vi "Counter+AOtest.vi"() -> ()   [LabVIEW 2010]
uses:
  <vilib>/DAQmx/write.llb/DAQmx Write (Analog 2D DBL NChan NSamp).vi
  <vilib>/DAQmx/read.llb/DAQmx Read (Counter 1D U32 1Chan NSamp).vi
  <vilib>/DAQmx/create/channels.llb/DAQmx Create Channel (CI-Count Edges).vi
  <vilib>/DAQmx/configure/timing.llb/DAQmx Timing (Sample Clock).vi
  <vilib>/DAQmx/create/channels.llb/DAQmx Create Channel (AO-Voltage-Basic).vi
  <vilib>/daqmx/miscellaneous.llb/DAQmx Fill In Error Info.vi
  Program Files/National Instruments/LabVIEW 2010/resource/objmgr/daqmx.rc
panel:
  out "counter 1":u32[](graph)
  out "counter 2":u32[](graph)
  out "Y waveform":dbl[](graph)
  out "X waveform":dbl[](graph)
  out "error out AO":errorcluster
  out "task out AO":refnum<k21>
  out "error out CH1":errorcluster
  out "error out CH2":errorcluster
  out "Task CI CH2":refnum<k21>
  out "Task CI CH1":refnum<k21>
  in  "Field Size(V)":i8=1 caption="x-res" min=0 max=10
  out "P":dbl
  out "AI number of scans":i32=423936
  out "bin value":u32=1 caption="length [ms]" min=1 max=8 step=1
  in  "AI rate":u32=100000
  out "y-res new":i32=128
  out "x-res new":i32=128 caption="x-res new]"
  in  "resolution":u16(ring)=512 items=["128x"=128, "256x"=256, "512x"=512, "1024x"=1024]
  in  "x-res":i32=128
  in  "y-res":i32=128 caption="y-res]"
  in  "quick res":bool caption="quick"
  out "Y-WaveArray":dbl[](array[numeric])
  out "X-WaveArray":dbl[](array[numeric])
  out "numPixels":dbl
  in  "AO rate":u32=100000
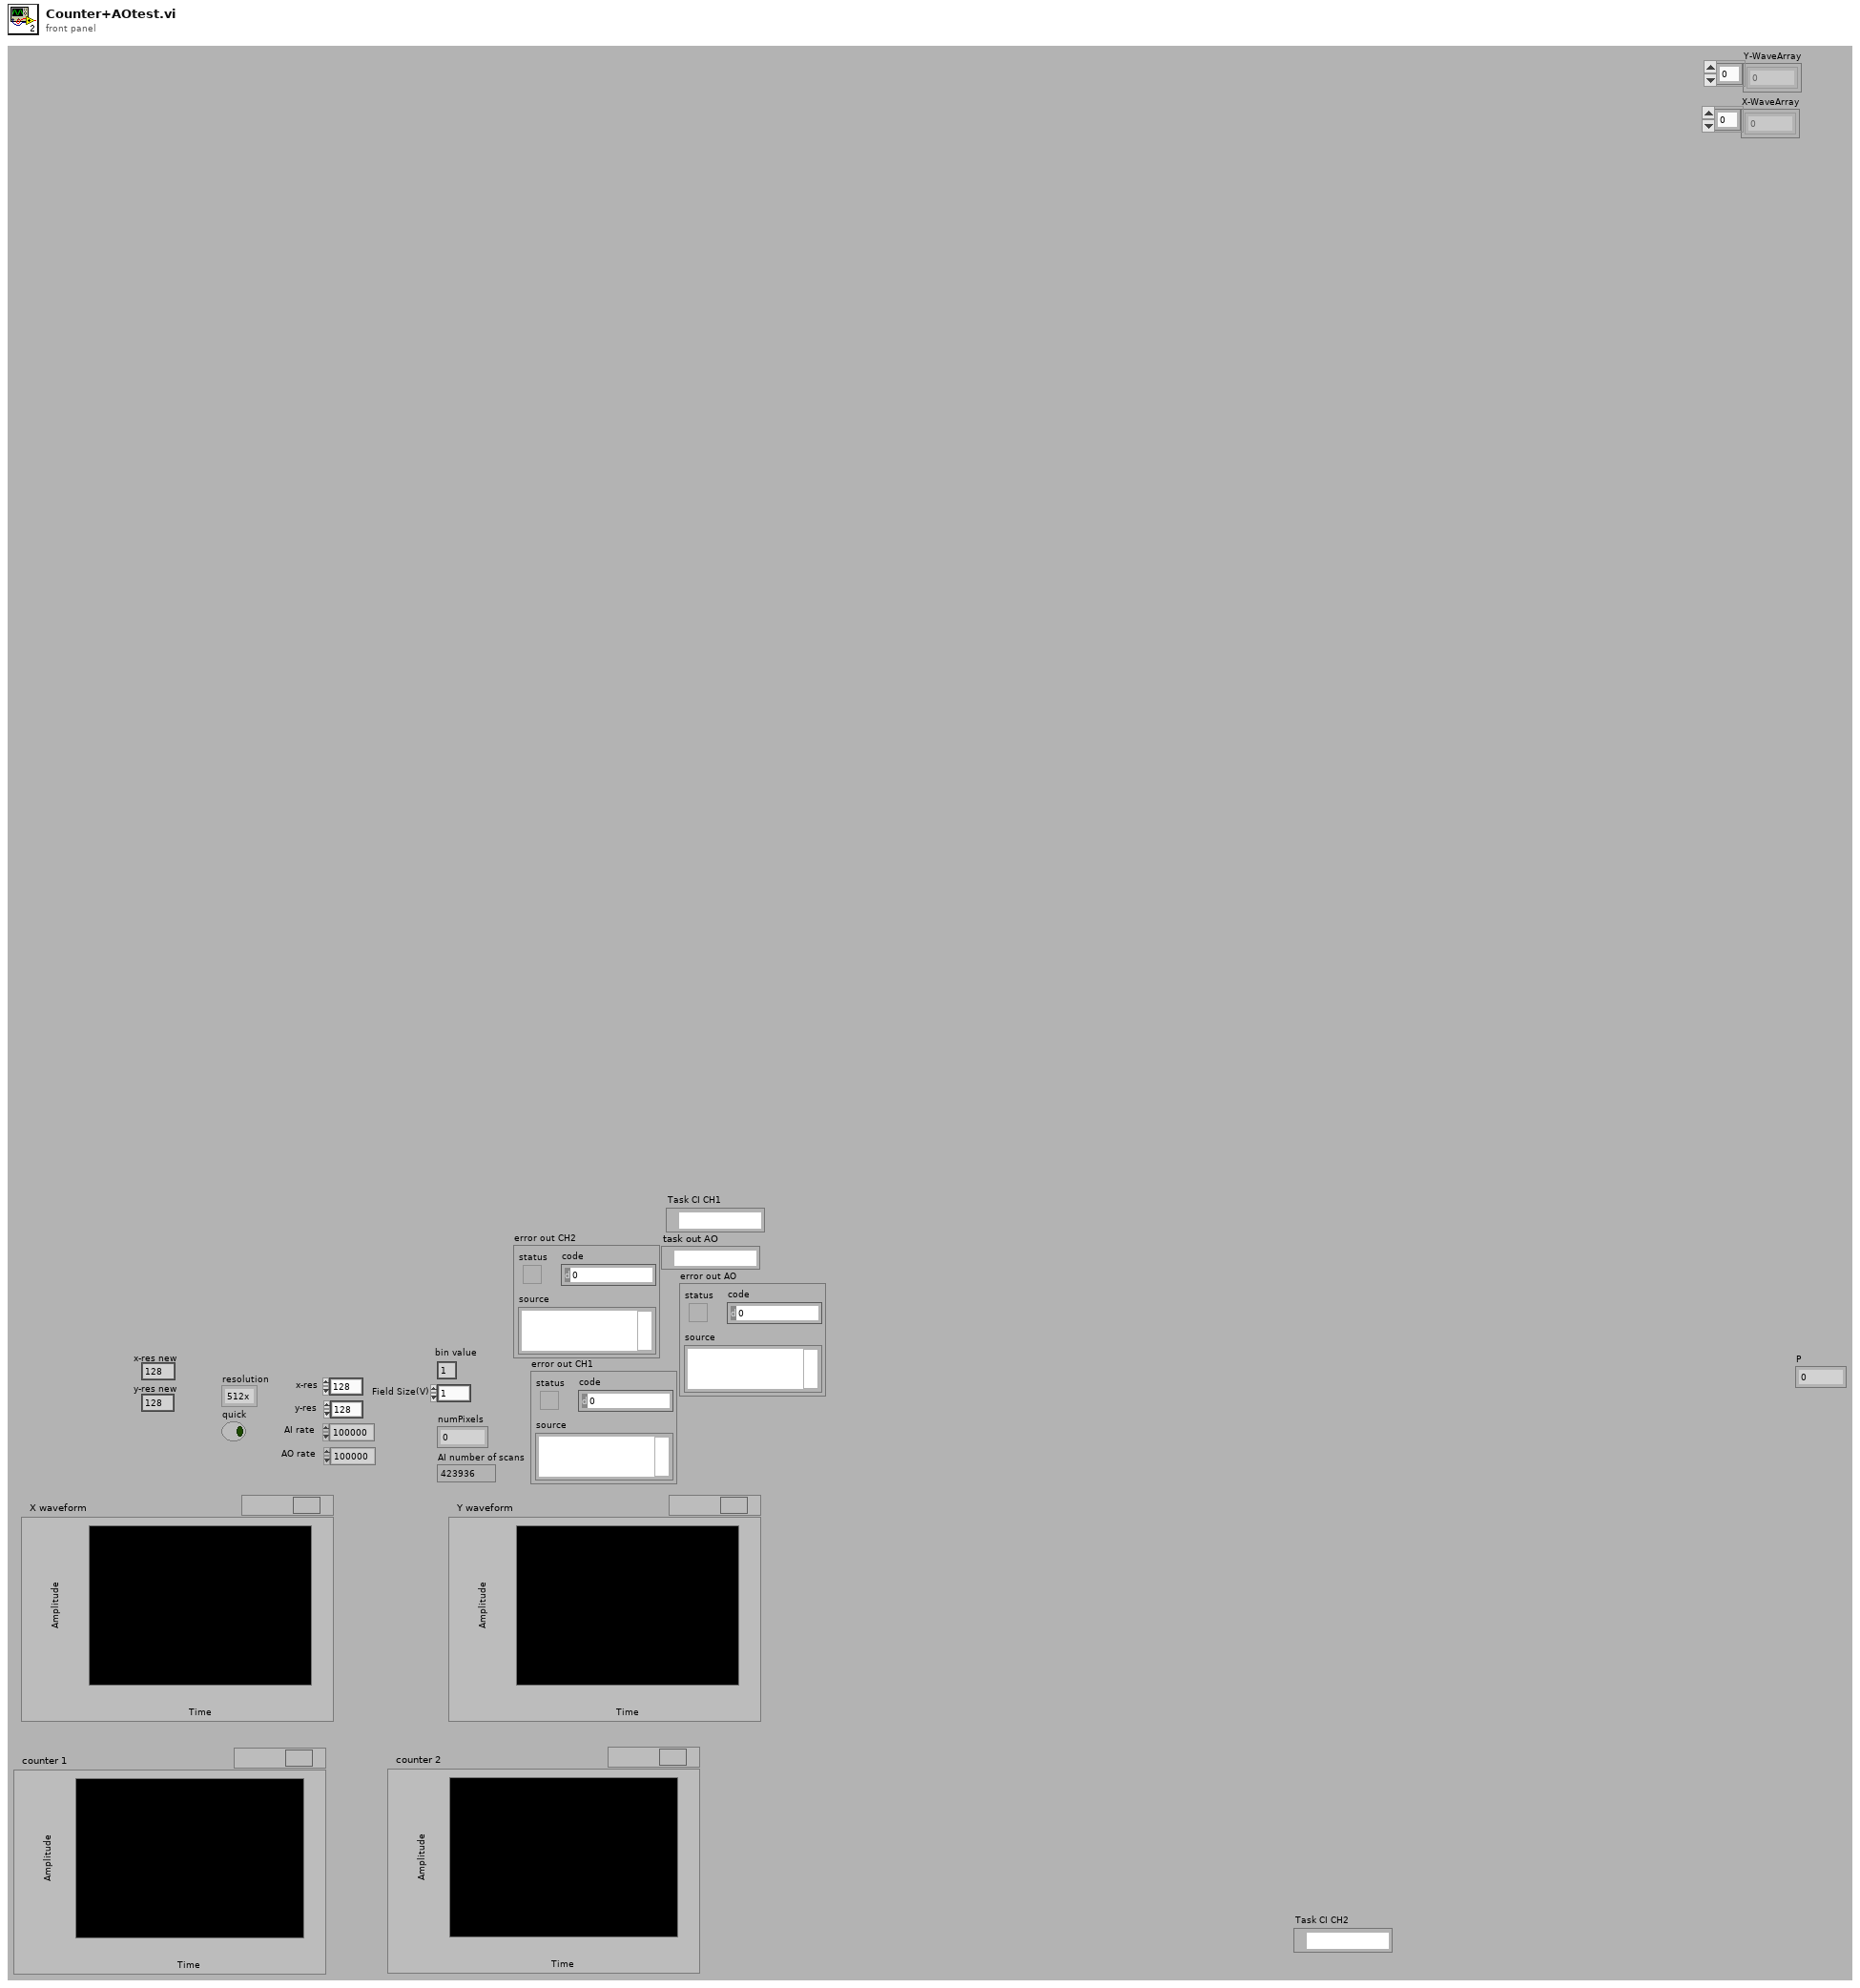
[diagram p1: front panel]
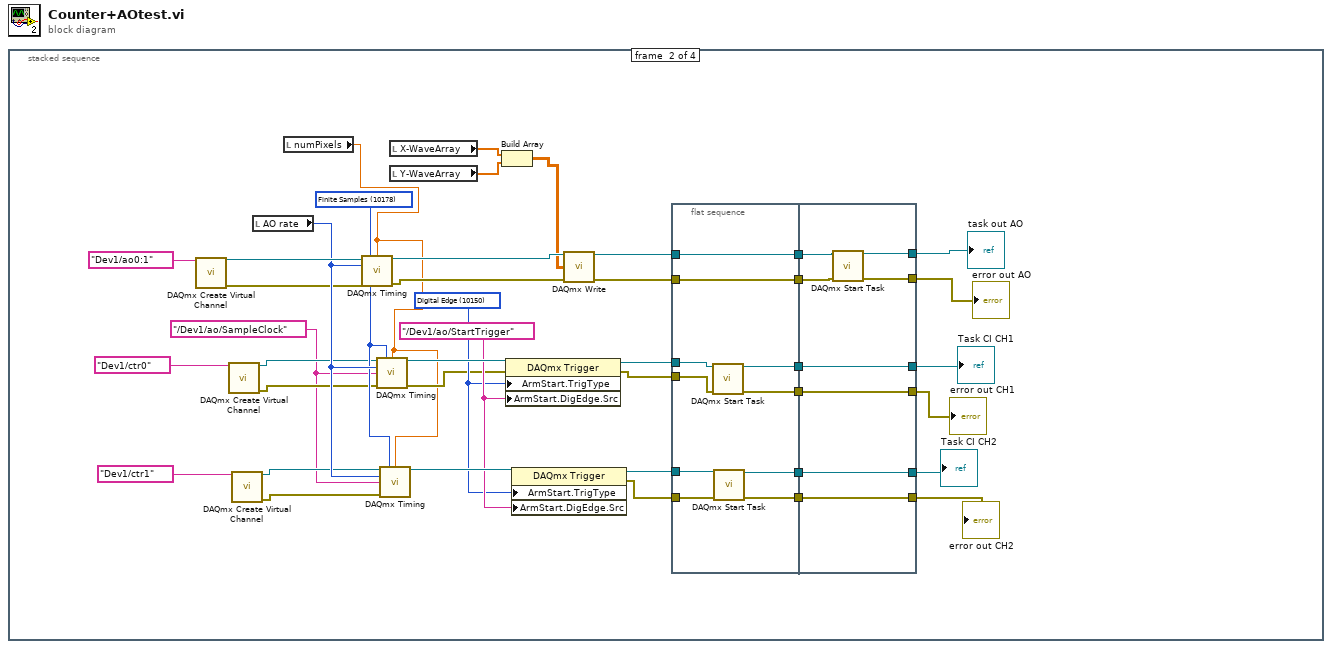
[diagram p0: block diagram]
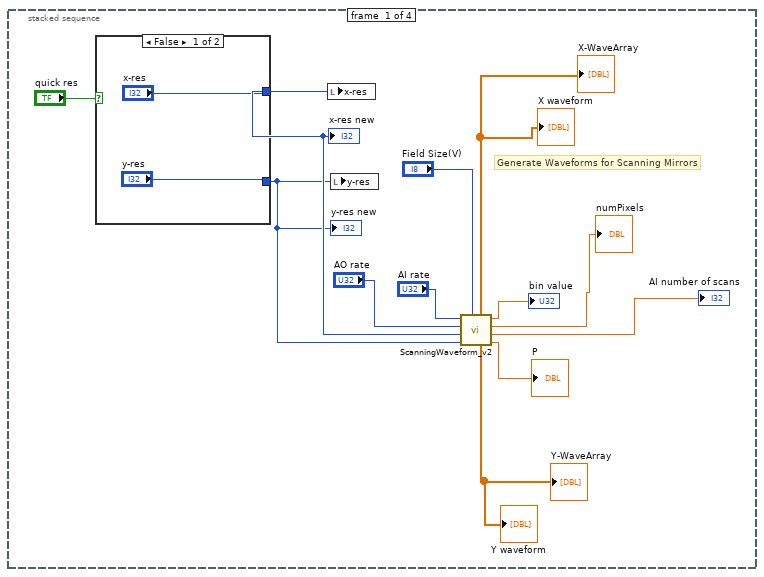
[diagram p2: hidden frame]
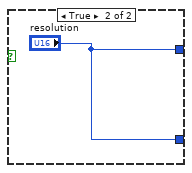
[diagram p3: hidden frame]
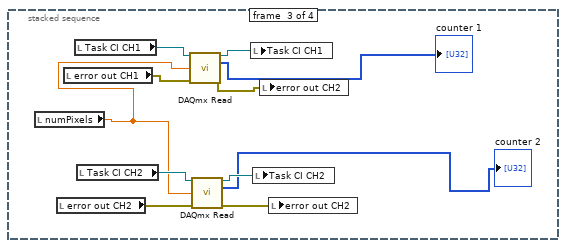
[diagram p4: hidden frame]
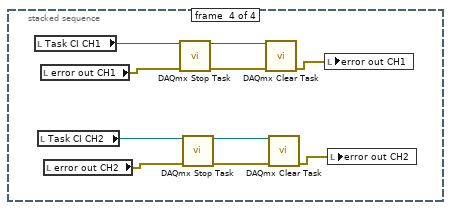
[diagram p5: hidden frame]
diagram:
  n1 = stacked-sequence {
    frame #0 {
      # "Generate Waveforms for Scanning Mirrors"
      n2 = case shown="False" "quick res" {
        tunnel: ["x-res" "resolution"] -> w10
        tunnel: ["y-res" "resolution"] -> w9
        frame False {
        }
        frame True {
        }
      }
      "x-res new" <- w10
      "y-res new" <- w9
      n3 = local write "x-res"(w10) -> ()
      n4 = local write "y-res"(w9) -> ()
      n5 = call "ScanningWaveform_v2.vi"("Vin"="Field Size(V)", "yPixels"=w9, "xPixels"=w10, "AOrate"="AO rate", "AIrate"="AI rate") -> ("P"=→"P":dbl, "numScan"=→"AI number of scans":dbl, "numPixels"=→"numPixels":dbl, "bin"=→"bin value":dbl, "Y-WaveArray"=→"Y-WaveArray" →"Y waveform":dbl[], "X-WaveArray"=→"X-WaveArray" →"X waveform":dbl[])  [unwired: 1 in]
    }
    frame #1 {
      w17 = tag "/Dev1/ao/SampleClock" ("source")
      w40 = 10150 items=["Digital Edge"=10150, "None"=10230] ("ArmStart.TrigType")
      w41 = tag "/Dev1/ao/StartTrigger" ("ArmStart.DigEdge.Src")
      w49 = 10178 items=["Finite Samples"=10178, "Continuous Samples"=10123, "Hardware Timed Single Point"=12522] ("sample mode")
      n6 = call-poly <vilib>:"DAQmx Create Virtual Channel.vi"("physical channels"=tag "Dev1/ao0:1") -> ("task out"=w53:refnum<k21>, "error out"=w46:errorcluster)  [unwired: 13 in]
      n7 = call-poly <vilib>:"DAQmx Create Virtual Channel.vi"("counter"=tag "Dev1/ctr0") -> ("task out"=w48:refnum<k21>, "error out"=w45:errorcluster)  [unwired: 13 in]
      n8 = call-poly <vilib>:"DAQmx Create Virtual Channel.vi"("counter"=tag "Dev1/ctr1") -> ("task out"=w47:refnum<k21>, "error out"=w44:errorcluster)  [unwired: 13 in]
      n9 = local read "AO rate"() -> (w50:u32)
      n10 = local read "numPixels"() -> (w16:dbl)
      n11 = call-poly <vilib>:"DAQmx Timing.vi"("task/channels in"=w53, "sample mode"=w49, "samples per channel"=w16, "rate"=w50, "error in"=w46) -> ("task out"=w34:refnum<k21>, "error out"=w30:errorcluster)  [unwired: 9 in]
      n12 = call-poly <vilib>:"DAQmx Timing.vi"("task/channels in"=w48, "sample mode"=w49, "samples per channel"=w16, "rate"=w50, "source"=w17, "error in"=w45) -> ("task out"=w43:refnum<k21>, "error out"=w39:errorcluster)  [unwired: 8 in]
      n13 = call-poly <vilib>:"DAQmx Timing.vi"("task/channels in"=w47, "sample mode"=w49, "samples per channel"=w16, "rate"=w50, "source"=w17, "error in"=w44) -> ("task out"=w42:refnum<k21>)  [unwired: 8 in, 1 out]
      n14 = local read "X-WaveArray"() -> (w32:dbl[])
      n15 = local read "Y-WaveArray"() -> (w33:dbl[])
      n16 = Build Array(w32, w33) -> (w31:dbl[][])
      n17 = property class="DAQmx Trigger"(reference=w43, error in=w39, "ArmStart.TrigType"=w40, "ArmStart.DigEdge.Src"=w41) -> (reference out=w38:refnum<k21>, error out=w37:errorcluster)
      n18 = property class="DAQmx Trigger"(reference=w42, "ArmStart.TrigType"=w40, "ArmStart.DigEdge.Src"=w41) -> (reference out=w36:refnum<k21>, error out=w35:errorcluster)  [unwired: 1 in]
      n19 = call-poly <vilib>:"DAQmx Write.vi"("task/channels in"=w34, "data"=w31, "error in"=w30) -> ("task out"=w28:refnum<k21>, "error out"=w29:errorcluster)  [unwired: 10 in, 1 out]
      n20 = flat-sequence {
        tunnel: w38 -> [w66]
        tunnel: w37 -> [w65]
        tunnel: w36 -> [w64]
        tunnel: w35 -> [w63]
        tunnel: [w62] -> w56
        tunnel: w29 -> [w62]
        tunnel: w28 -> [w61]
        tunnel: [w61] -> w55
        tunnel: [w60] -> w27
        tunnel: [w59] -> w25
        tunnel: [w58] -> w23
        tunnel: [w57] -> w22
        tunnel: w56 -> [w74]
        tunnel: w55 -> [w73]
        tunnel: [w72] -> w19
        tunnel: [w71] -> w26
        tunnel: w27 -> [w71]
        tunnel: w25 -> [w70]
        tunnel: [w70] -> w24
        tunnel: w23 -> [w69]
        tunnel: [w69] -> w20
        tunnel: w22 -> [w68]
        tunnel: [w68] -> w21
        tunnel: [w67] -> w18
        frame #0 {
          n21 = call <vilib>:"DAQmx Start Task.vi"("task/channels in"=w66, "error in"=w65) -> ("task out"=w60:refnum<k21>, "error out"=w58:errorcluster)  [unwired: 12 in]
          n22 = call <vilib>:"DAQmx Start Task.vi"("task/channels in"=w64, "error in"=w63) -> ("task out"=w59:refnum<k21>, "error out"=w57:errorcluster)  [unwired: 12 in]
        }
        frame #1 {
          n23 = call <vilib>:"DAQmx Start Task.vi"("task/channels in"=w73, "error in"=w74) -> ("task out"=w72:refnum<k21>, "error out"=w67:errorcluster)  [unwired: 12 in]
        }
      }
      "Task CI CH1" <- w26
      "Task CI CH2" <- w24
      "error out CH2" <- w21
      "error out CH1" <- w20
      "task out AO" <- w19
      "error out AO" <- w18
    }
    frame #2 {
      n24 = local read "numPixels"() -> (w77:dbl)
      n25 = local read "error out CH2"() -> (w80:errorcluster)
      n26 = local read "error out CH1"() -> (w81:errorcluster)
      n27 = local read "Task CI CH1"() -> (w85:refnum<k21>)
      n28 = local read "Task CI CH2"() -> (w82:refnum<k21>)
      n29 = call-poly <vilib>:"DAQmx Read.vi"("task/channels in"=w85, "number of samples per channel"=w77, "error in"=w81) -> ("task out"=w84:refnum<k21>, "data"=→"counter 1":u32[], "error out"=w76:errorcluster)  [unwired: 10 in]
      n30 = call-poly <vilib>:"DAQmx Read.vi"("task/channels in"=w82, "number of samples per channel"=w77, "error in"=w80) -> ("task out"=w83:refnum<k21>, "data"=→"counter 2":u32[], "error out"=w79:errorcluster)  [unwired: 10 in]
      n31 = local write "Task CI CH1"(w84) -> ()
      n32 = local write "Task CI CH2"(w83) -> ()
      n33 = local write "error out CH2"(w76) -> ()
      n34 = local write "error out CH2"(w79) -> ()
    }
    frame #3 {
      n35 = local read "Task CI CH1"() -> (w94:refnum<k21>)
      n36 = local read "Task CI CH2"() -> (w87:refnum<k21>)
      n37 = local read "error out CH1"() -> (w93:errorcluster)
      n38 = local read "error out CH2"() -> (w88:errorcluster)
      n39 = call <vilib>:"DAQmx Stop Task.vi"("task/channels in"=w94, "error in"=w93) -> ("task out"=w95:refnum<k21>, "error out"=w92:errorcluster)  [unwired: 12 in]
      n40 = call <vilib>:"DAQmx Stop Task.vi"("task/channels in"=w87, "error in"=w88) -> ("task out"=w86:refnum<k21>, "error out"=w89:errorcluster)  [unwired: 12 in]
      n41 = call <vilib>:"DAQmx Clear Task.vi"("task in"=w95, "error in"=w92) -> ("error out"=w91:errorcluster)  [unwired: 13 in]
      n42 = call <vilib>:"DAQmx Clear Task.vi"("task in"=w86, "error in"=w89) -> ("error out"=w90:errorcluster)  [unwired: 13 in]
      n43 = local write "error out CH1"(w91) -> ()
      n44 = local write "error out CH2"(w90) -> ()
    }
  }
